vi "Yscalingtest.vi"(6 "current":dbl, 8 "Nano Z Read":dbl, 9 "Current Maxed?":bool, 10 "Y":dbl, 11 "Plane Height":dbl) -> (3 "y scaled":dbl, 4 "Testoutput":dbl)   [LabVIEW 2017]
uses:
  <userlib>/HapticSTM/Feedbackless - Testdata/Yscalingtest Folder/HapticSTM.lvlib
panel:
  out "current":cluster{"current":dbl}(graph)
  out "Zpos":T1(graph)
  out "appended array":dbl[](array[numeric])
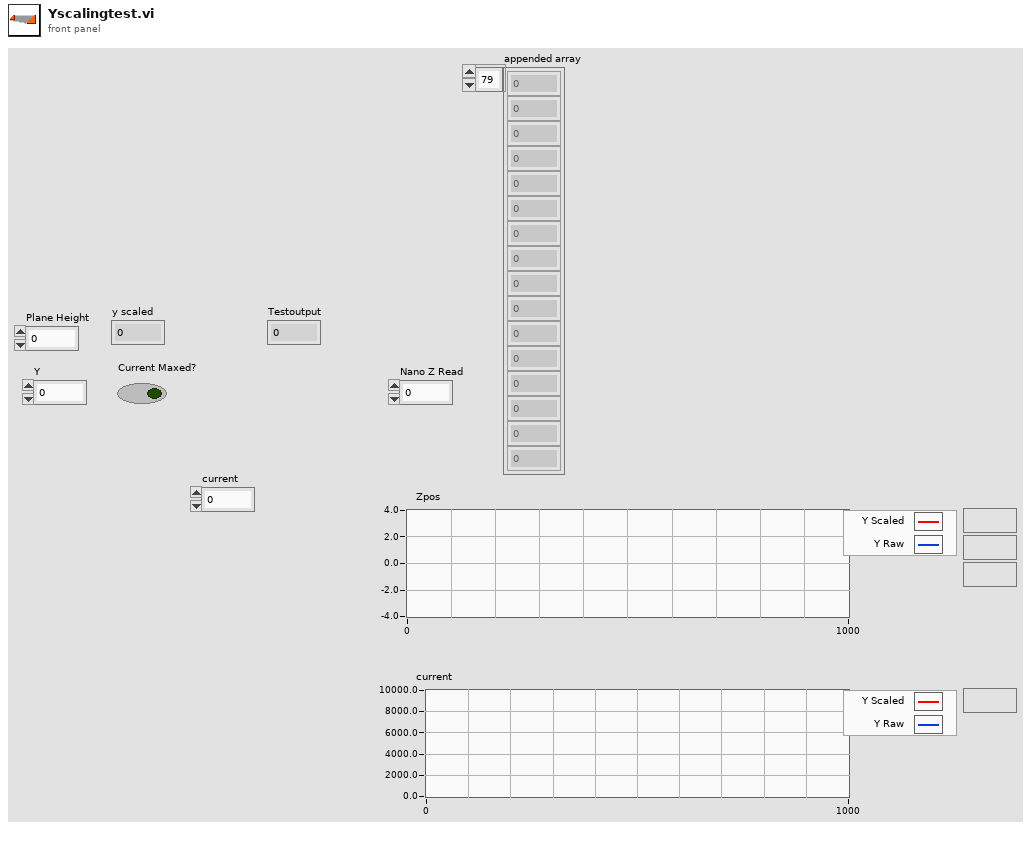
[diagram p1: front panel]
types:
  T1 = cluster{dbl, "function return":dbl, "function return":dbl}
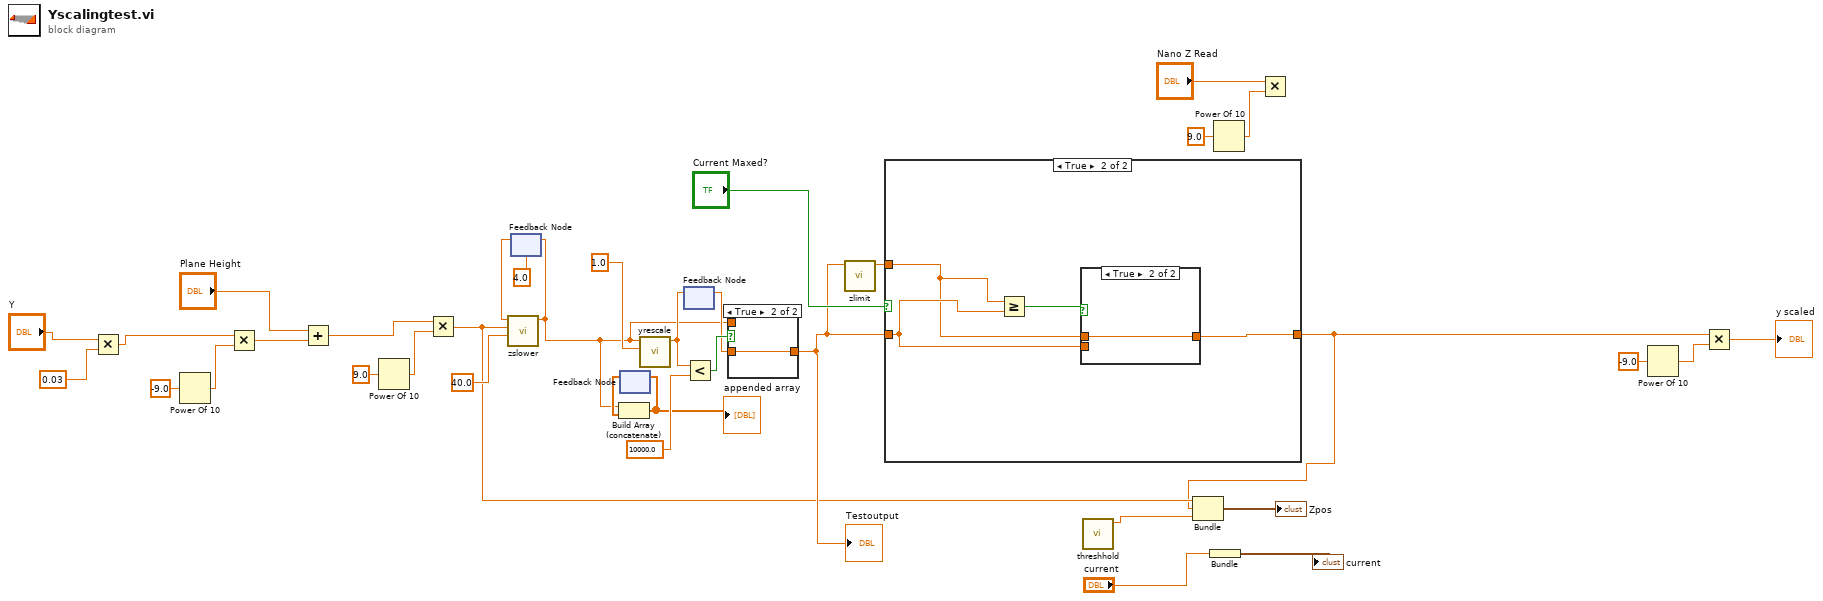
[diagram p0: block diagram]
diagram:
  n1 = Multiply(x="Y", y=0.03) -> (x*y=w32:dbl)
  n2 = Power Of 10(x=-9.0) -> (10^x=w31:dbl)
  n3 = Multiply(x=w32, y=w31) -> (x*y=w33:dbl)
  n4 = Add(x="Plane Height", y=w33) -> (x+y=w36:dbl)
  n5 = Power Of 10(x=9.0) -> (10^x=w35:dbl)
  n6 = Multiply(x=w36, y=w35) -> (x*y=w6:dbl)
  n7 = feedback #1(4.0 ("function return")) -> (w9:dbl)
  n8 = call <userlib>:"zslower.vi"("maxvel"=40.0, "labview_zpos_write"=w6, "nanonis_zpos_read"=w9) -> ("function return"=w8:dbl)  [unwired: 8 in]
  n9 = feedback-in #1(w8) -> ()
  n10 = feedback #2() -> (w11:dbl[])  [unwired: 1 in]
  n11 = Build Array (concatenate)(w8, w11) -> (w12:dbl[])
  "appended array" <- w12
  n12 = feedback-in #2(w12) -> ()
  n13 = call <userlib>:"yrescale.vi"("scalingfactor"=1.0, "ylabview"=w8) -> ("function return"=w17:dbl)  [unwired: 9 in]
  n14 = feedback-in #3(w17) -> ()
  n15 = feedback #3() -> (w16:dbl)  [unwired: 1 in]
  n16 = Less?(x=w17, y=10000.0) -> (x < y?=w18:bool)
  n17 = case shown="True" w18 {
    tunnel: [w37 w38] -> w20
    tunnel: w16 -> [_ w38]
    tunnel: w8 -> [w37 _]
    frame False {
    }
    frame True {
    }
  }
  "Testoutput" <- w20
  n18 = call <userlib>:"zlimit.vi"("yscaledinput"=w20) -> ("function return"=w21:dbl)  [unwired: 10 in]
  n19 = case shown="True" "Current Maxed?" {
    tunnel: [w39 w43] -> w5
    tunnel: w20 -> [w39 w41]
    tunnel: w21 -> [_ w40]
    frame False {
    }
    frame True {
      n20 = Greater Or Equal?(x=w40, y=w41) -> (x >= y?=w42:bool)
      n21 = case shown="True" w42 {
        tunnel: w40 -> [_ w45]
        tunnel: [w44 w45] -> w43
        tunnel: w41 -> [w44 _]
        frame False {
        }
        frame True {
        }
      }
    }
  }
  n22 = call <userlib>:"threshhold.vi"() -> ("function return"=w3:dbl)  [unwired: 11 in]
  n23 = Bundle(w6, "function return"=w5, "function return"=w3) -> (→"Zpos":T1)  [unwired: 1 in]
  n24 = Bundle("current"="current") -> (→"current":cluster{"current":dbl})  [unwired: 1 in]
  n25 = Power Of 10(x=9.0) -> (10^x=w15:dbl)
  n26 = Multiply(x="Nano Z Read", y=w15) -> ()  [unwired: 1 out]
  n27 = Power Of 10(x=-9.0) -> (10^x=w24:dbl)
  n28 = Multiply(x=w5, y=w24) -> (x*y=→"y scaled":dbl)
